vi "_USB_Close.vi"(8 "Error In":errorcluster) -> (0 "Error Out":errorcluster)   [LabVIEW 2020, in "MT_API.lvlib"]
doc: "MT_API INT32 __stdcall MT_Close_USB(void);"
uses:
  MT_API.lvlib
  MT_API_64.dll
panel:
  out "函数返回值":i32
  # "关闭设备的USB端口"
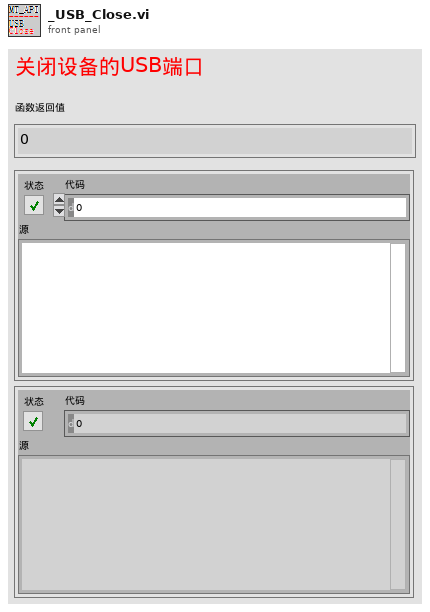
[diagram p1: front panel]
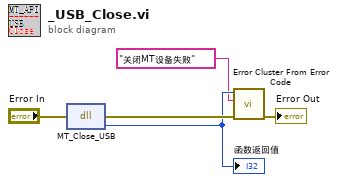
[diagram p0: block diagram]
diagram:
  n1 = dll-call lib="D:/Project NJU/lib/MT/MT_API_64.*" fn="MT_Close_USB"(error in="Error In") -> (error out=w3:errorcluster, "return type"=w2:i32)  [unwired: 2 in, 1 out]
  "函数返回值" <- w2
  n2 = call <vilib>:"Error Cluster From Error Code.vi"("error in (no error)"=w3, "error message (\"\")"="关闭MT设备失败", "error code (0)"=w2) -> ("error out"=→"Error Out":errorcluster)  [unwired: 6 in]
